vi "ORP电极校准.vi"() -> ()   [LabVIEW 2016, in "斯坦道多参数.lvlib"]
uses:
  <vilib>/Utility/miscctls.llb/LVPointTypeDef.ctl
  <vilib>/Analysis/NI_AALBase.lvlib
  <vilib>/Utility/config.llb/NI_LVConfig.lvlib
panel:
  in  "刷新按钮":bool
  out "第二点信号值":dbl
  out "第一点信号值":dbl
  out "通讯状态":string
  out "温度":dbl format="%#.2f"
  out "当前信号值":dbl caption="信号值" format="%#.2f"
  in  "校准停止":bool
  in  "校准启动":bool
  out "波形图表":dbl(graph) caption="历史曲线"
  out "第二点校准值":dbl
  out "第一点校准值":dbl
  in  "校准模式":u16(ring) items=["单点校准"]
  out "提示":string
  out "最小值":sgl format="%#.2f"
  out "最大值":sgl format="%#.2f"
  out "mean":dbl caption="均值" format="%#.2f"
  out "standard deviation":dbl caption="标准差" format="%#.2f"
  out "变异系数":dbl format="%#.6f"
  in  "标液1":dbl
  out "当前读取值":dbl caption="测量值" format="%#.2f"
  out "ORP偏移修正值":dbl format="%#.2f"
  # "ORP电极设定"
  # "请选择校准模式:"
  # "℃"
  # "mV"
  # "mV"
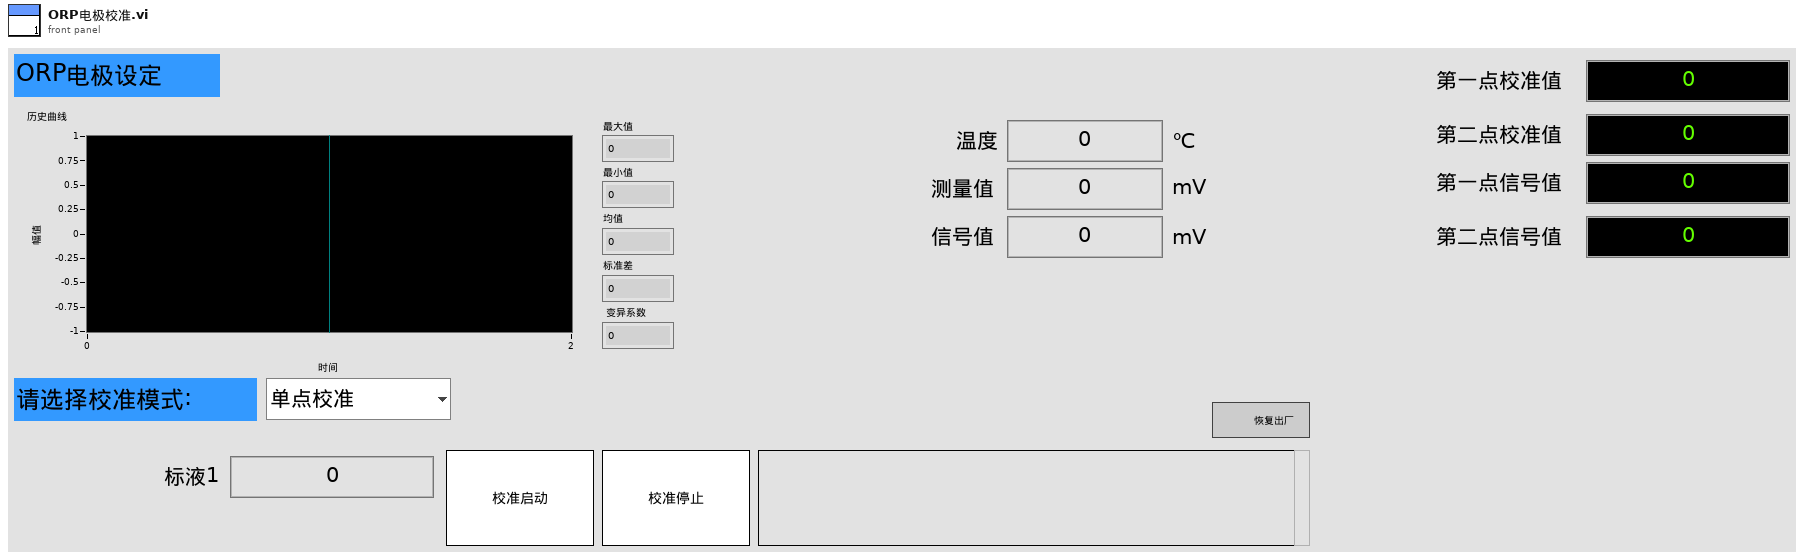
[diagram p1: front panel]
types:
  T1 = typedef "LVPointTypeDef.ctl" = cluster{"Horizontal":i16, "Vertical":i16}
  T2 = typedef "NI_LVConfig.lvlib/Config Data RefNum.ctl" = refnum<k1>
  T3 = cluster{"电极状态标志":u16, "电极型号标志":u16, "测量值":sgl, "温度测量值":sgl, "信号值":sgl, "温度信号值":sgl, "000AH_NC":sgl, "偏移修正值":sgl, "温度偏移修正值":sgl, "手动温度补偿值":sgl, "命令滤波设定":u16, "温度模式":enum16{"ATC", "MTC"}, "生产批次":u16, "传感器序号":u16, "串口地址":u16, "串口波特率":enum16{"9600", "19200", "115200"}, "串口校验位":enum16{"NONE", "ODD", "EVEN"}, "串口停止位":enum16{"1bit", "2bit"}}
  T4 = enum8{"Enabled", "Disabled", "Disabled and Grayed Out"}
  T5 = cluster{"ph":bool, "DO":bool, "Cond":bool, "Turb":bool, "叶绿素a":bool, "藻密度":bool, "ORP":bool}
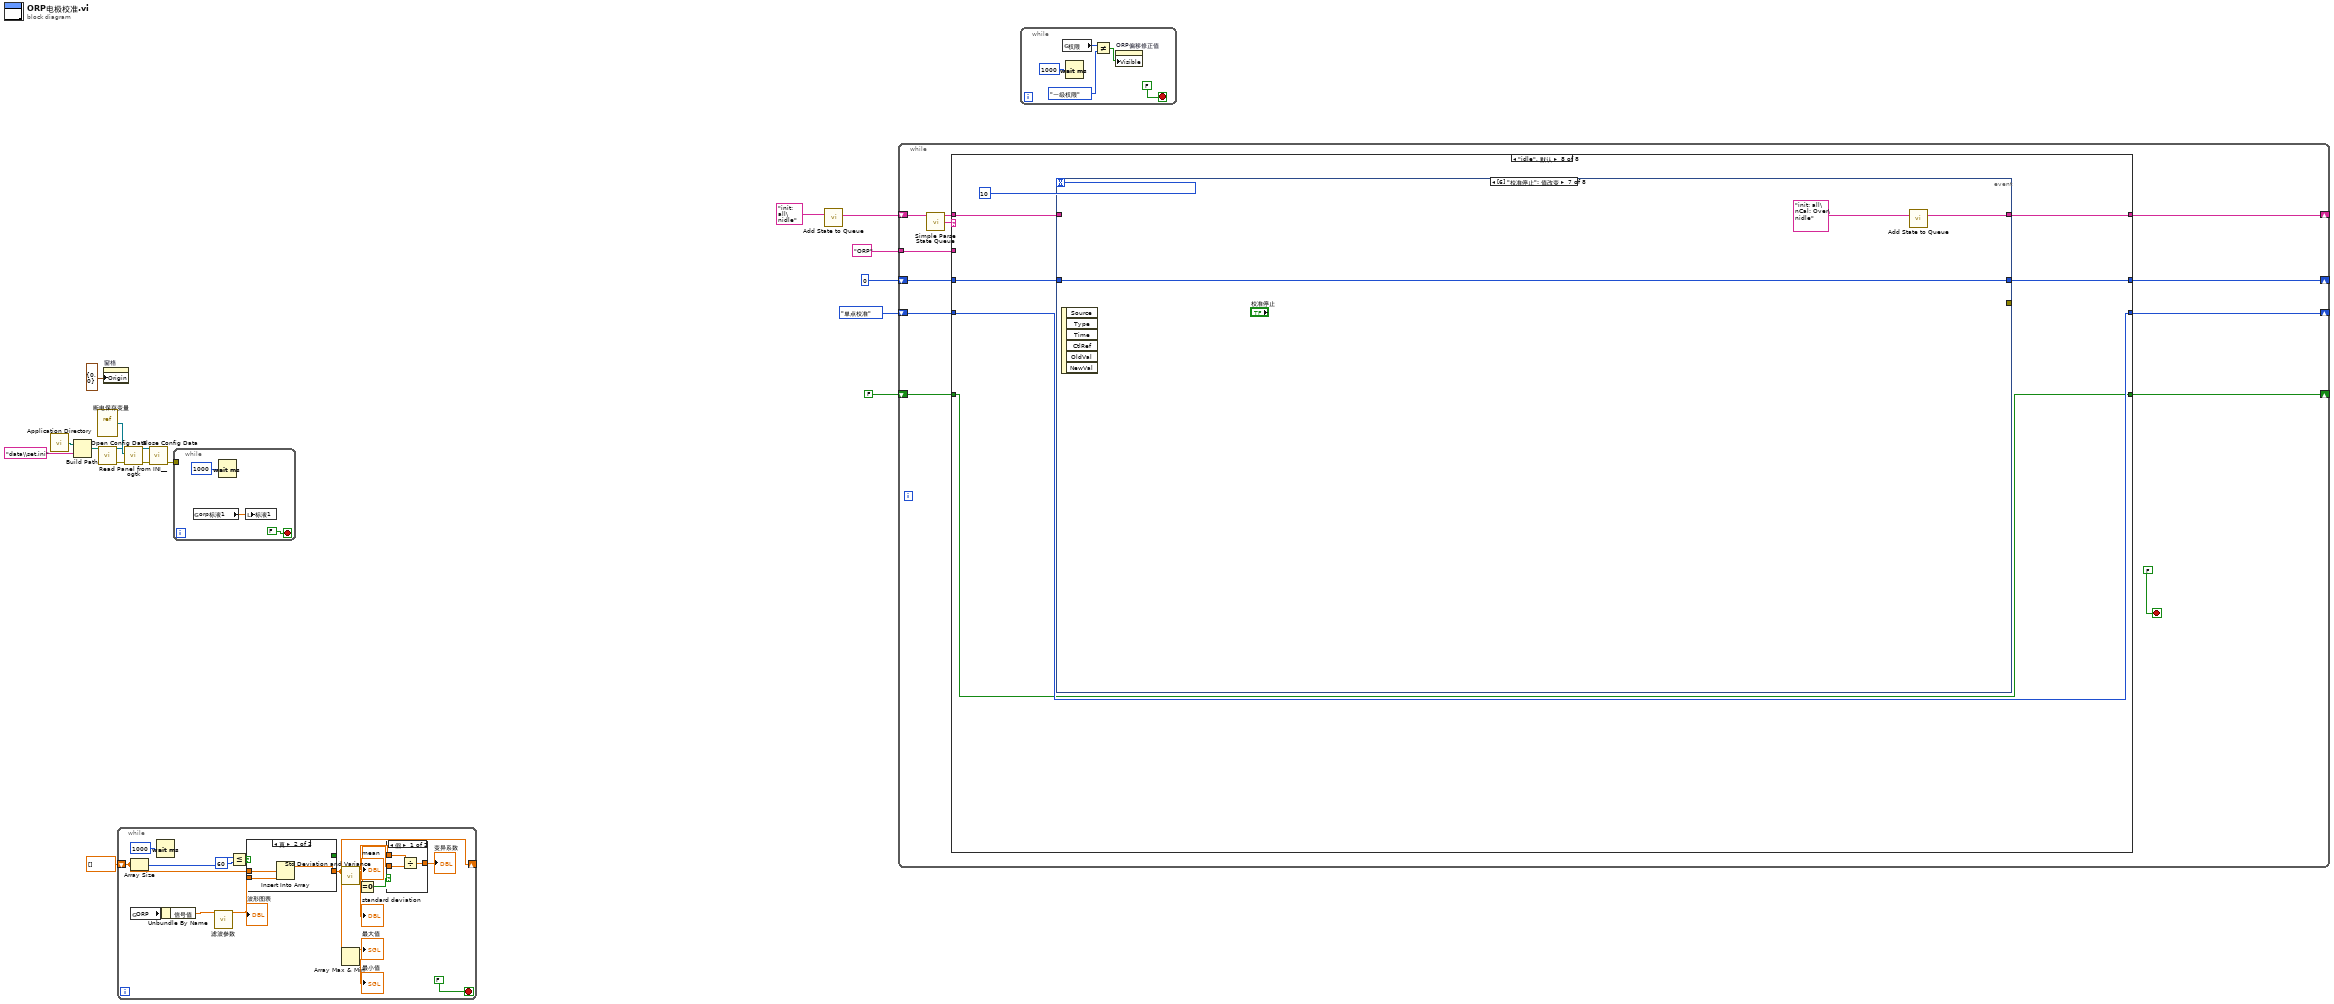
[diagram p0: block diagram]
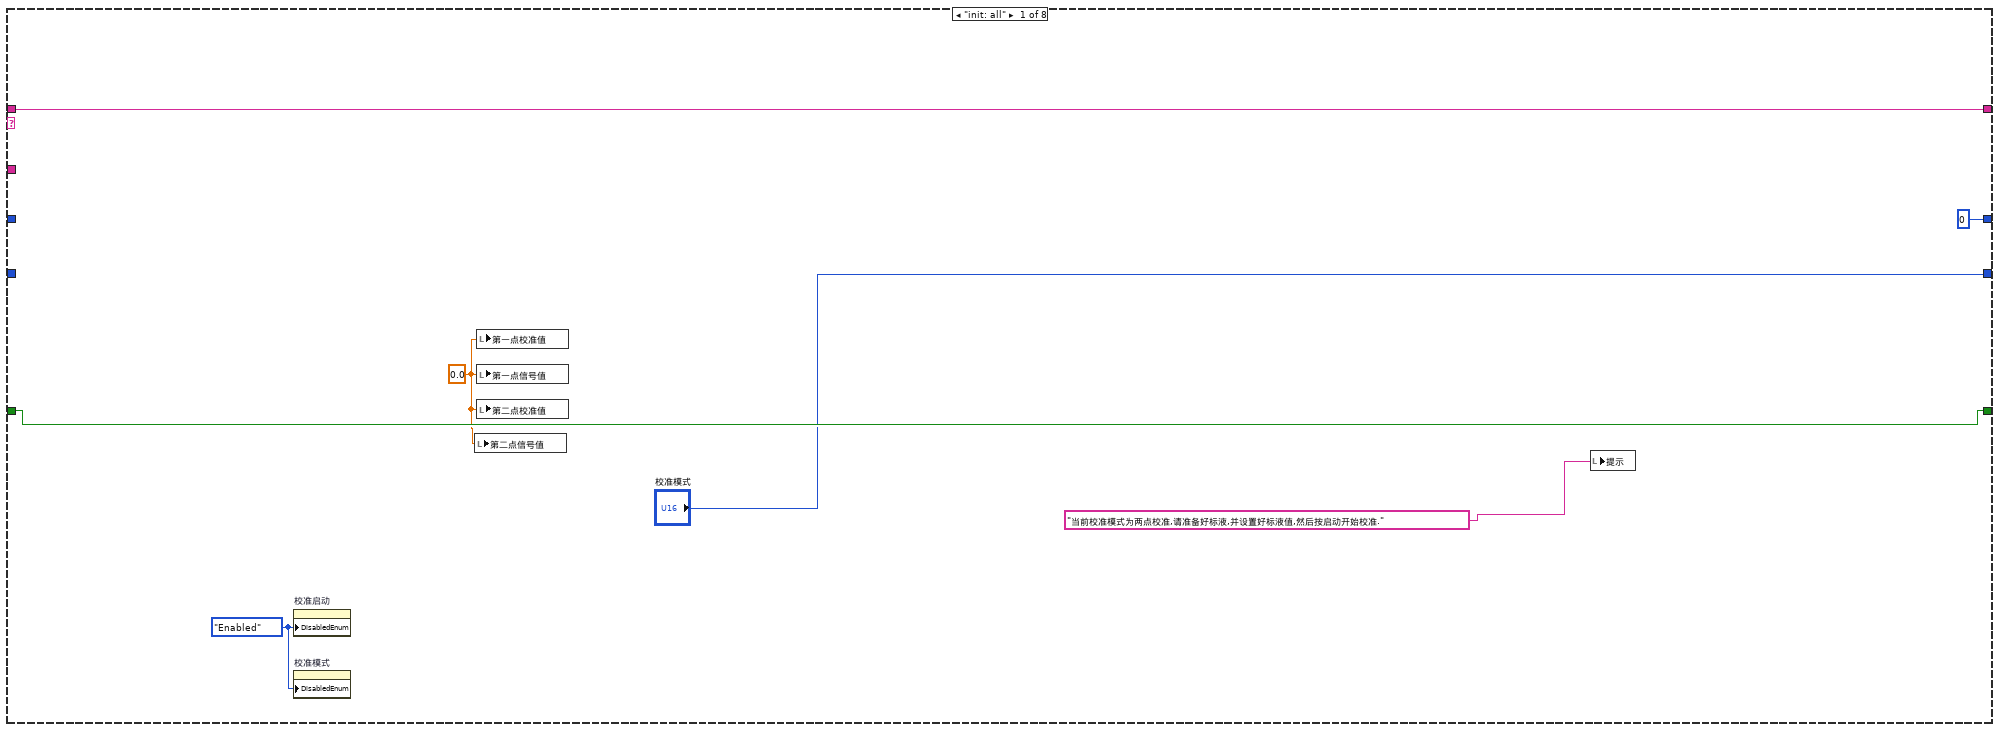
[diagram p2: hidden frame]
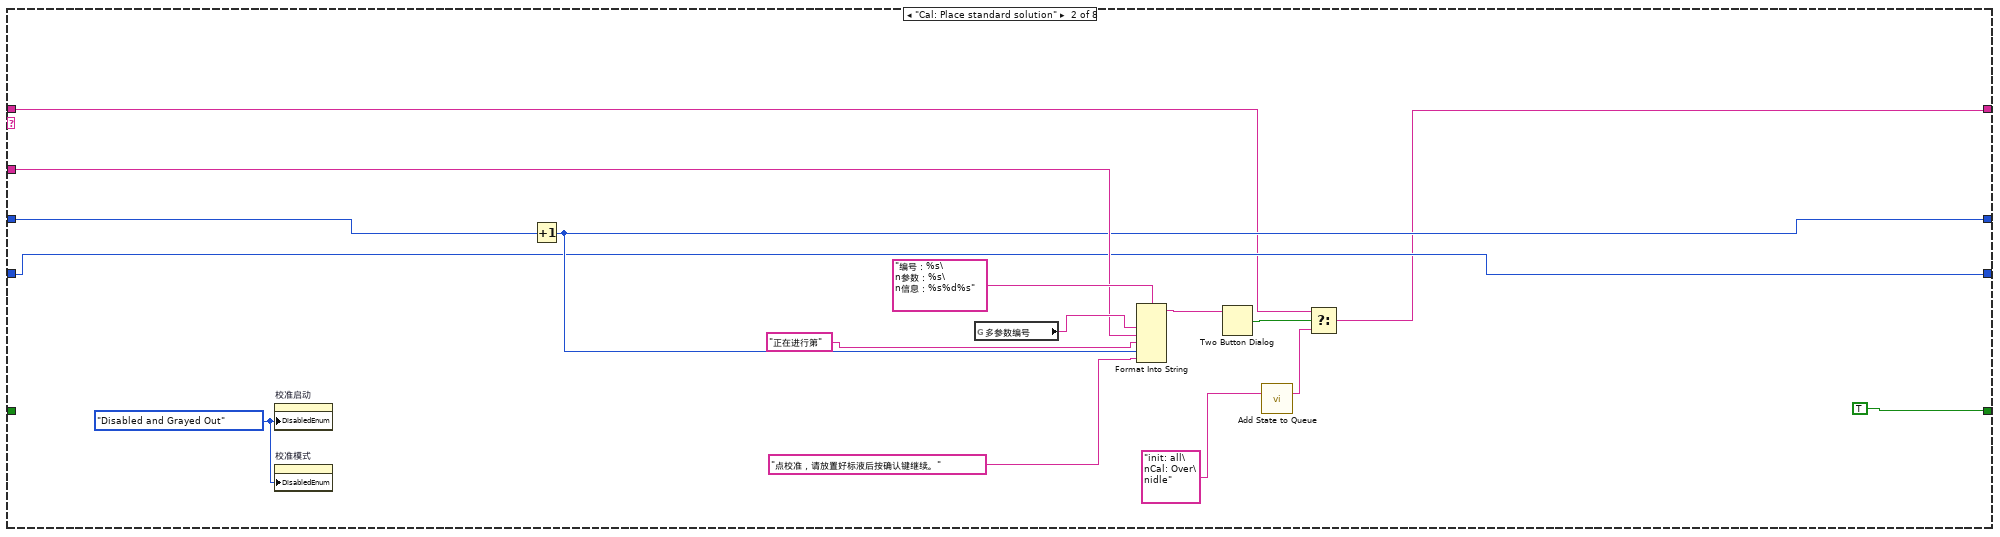
[diagram p3: hidden frame]
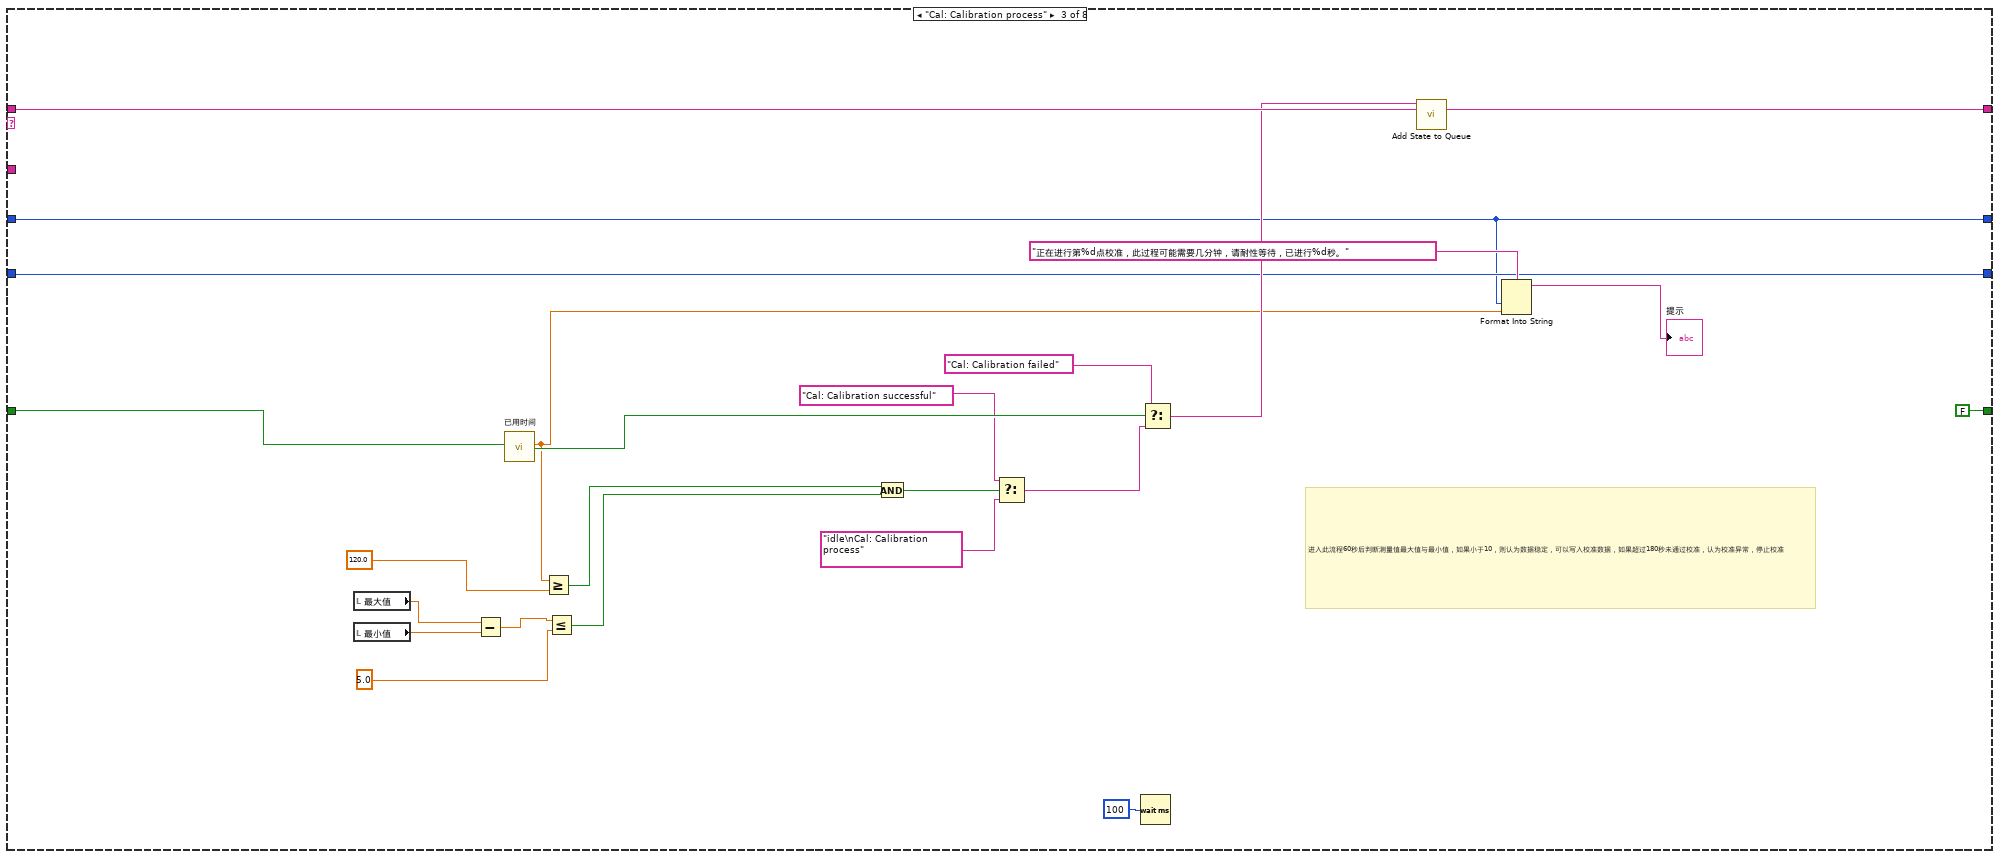
[diagram p4: hidden frame]
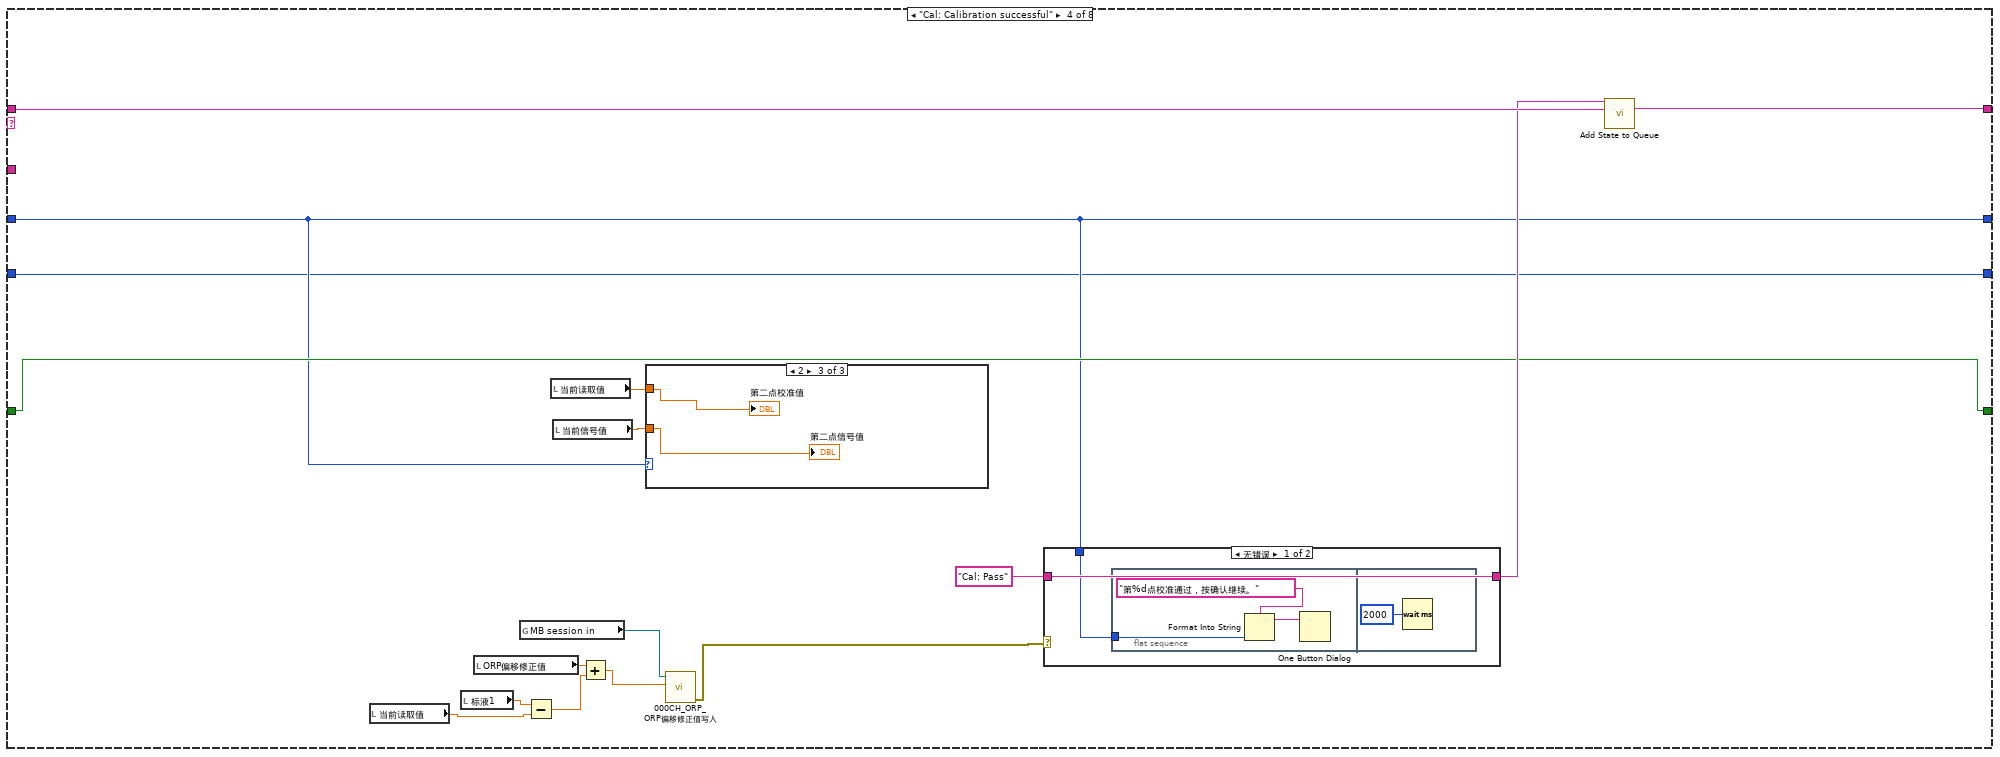
[diagram p5: hidden frame]
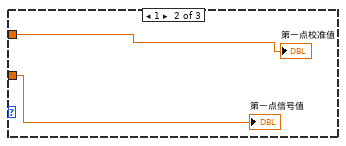
[diagram p7: hidden frame]
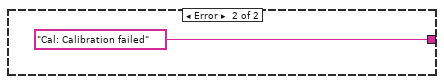
[diagram p8: hidden frame]
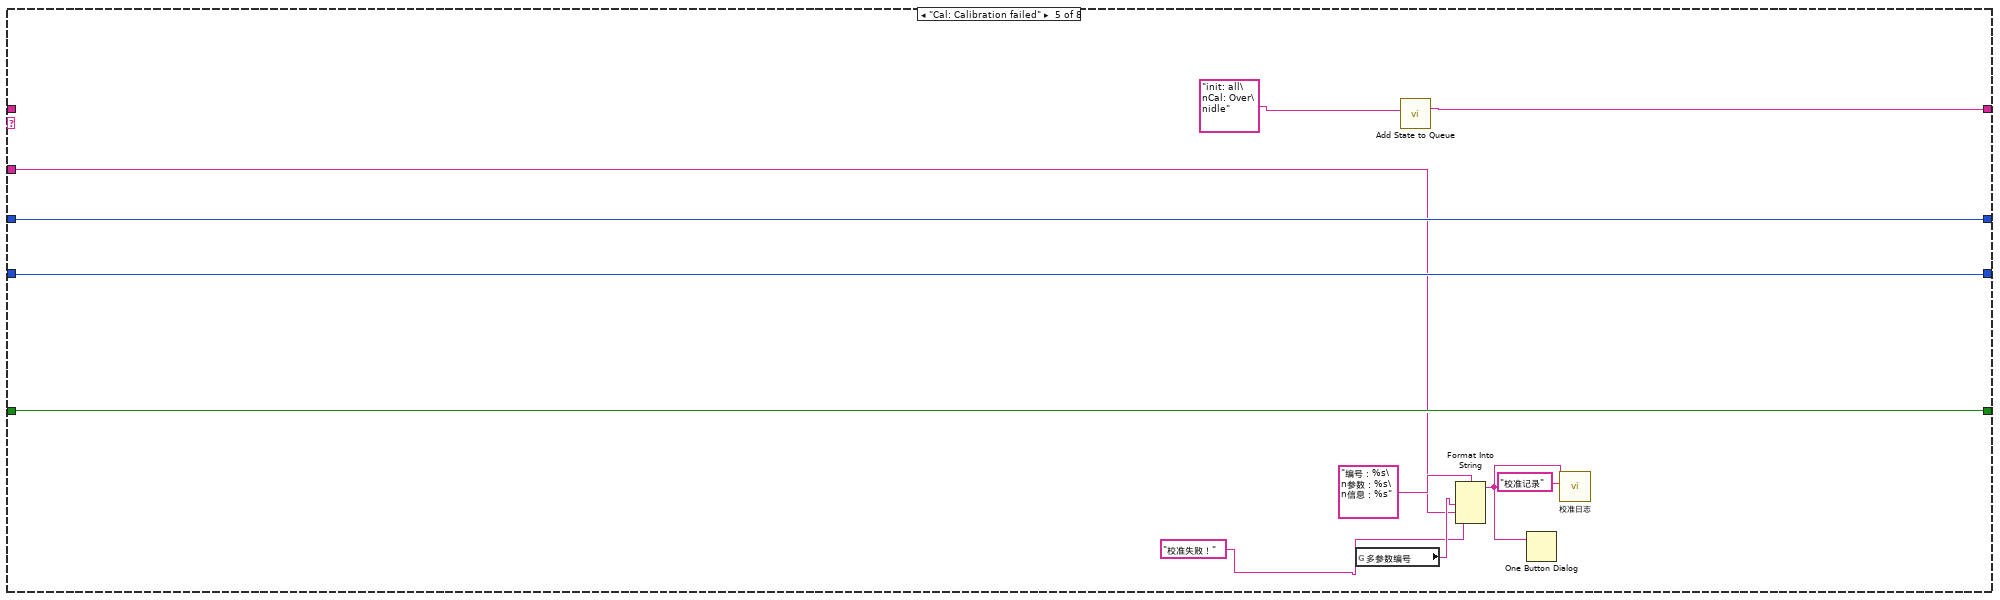
[diagram p9: hidden frame]
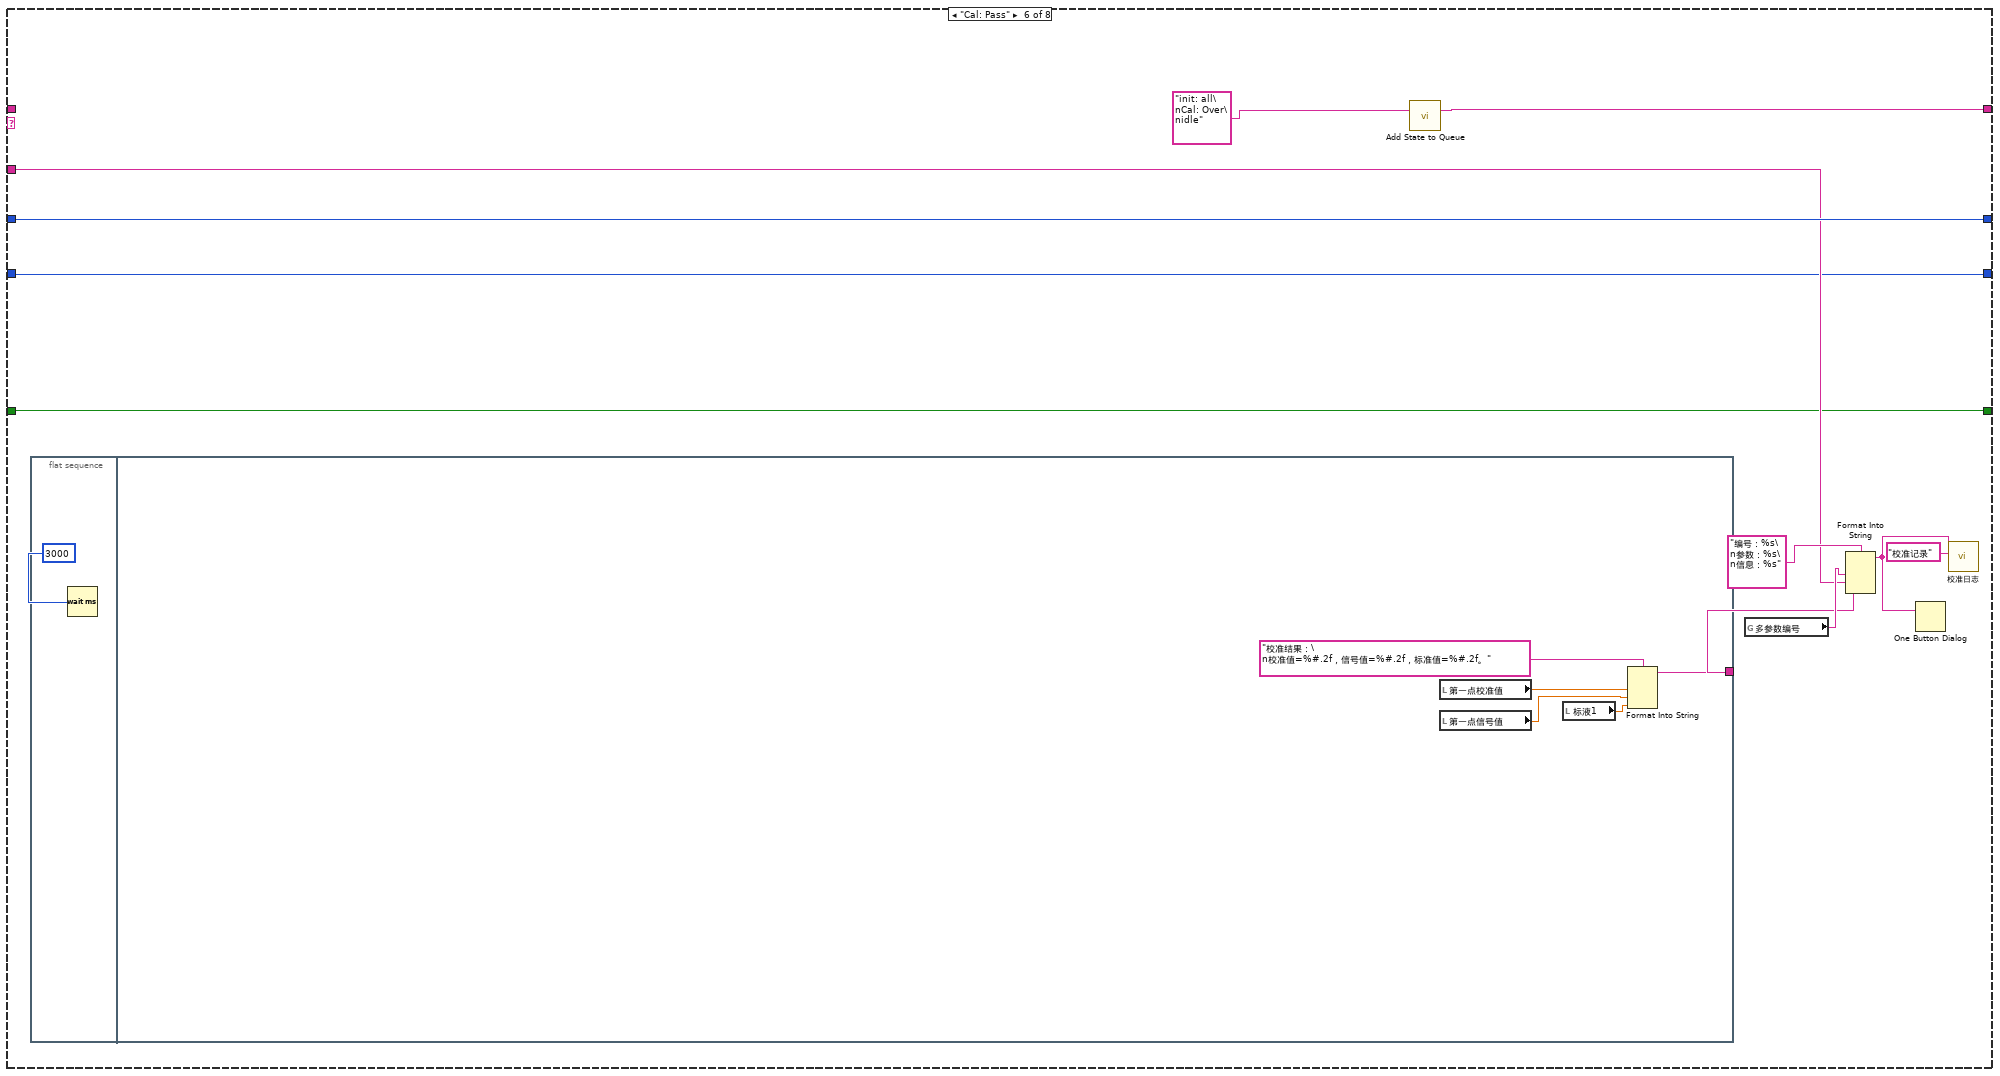
[diagram p10: hidden frame]
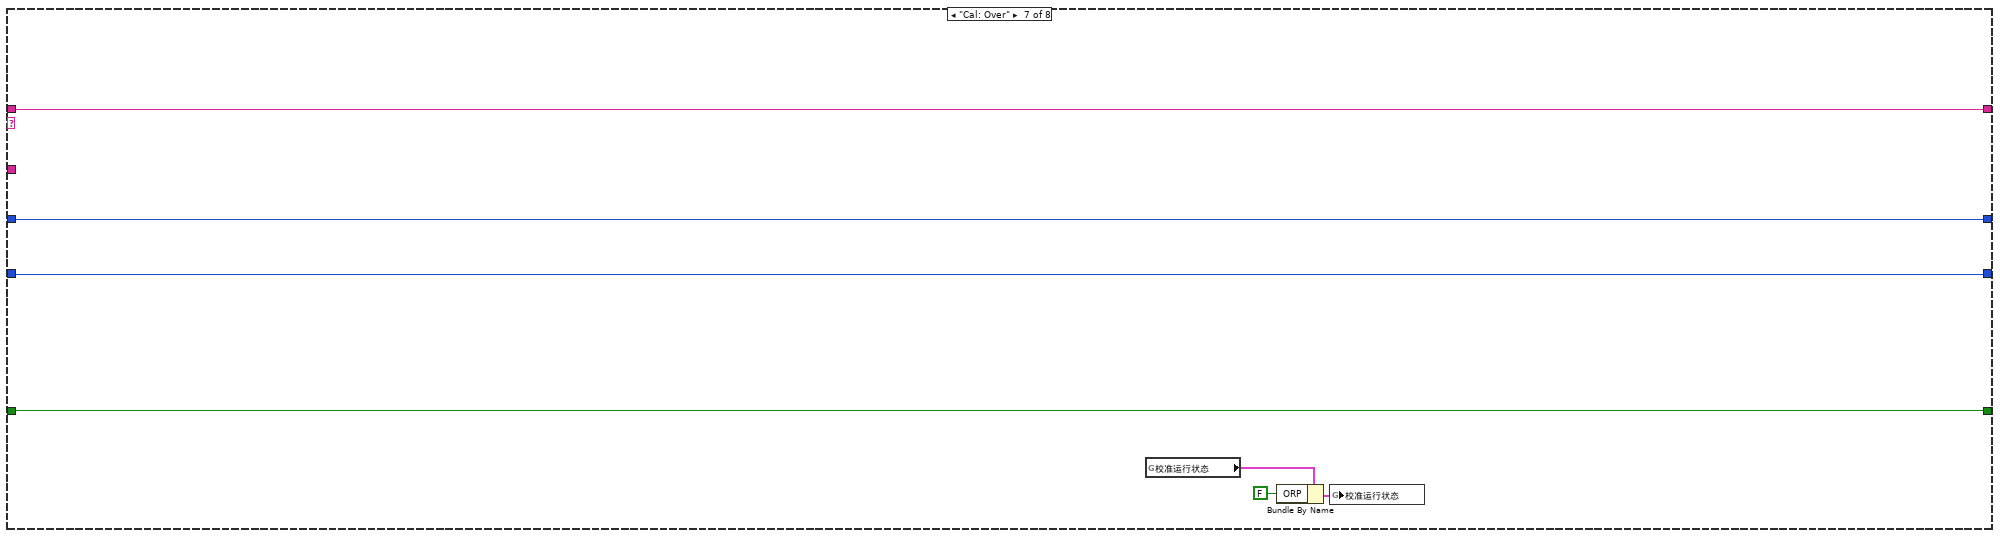
[diagram p11: hidden frame]
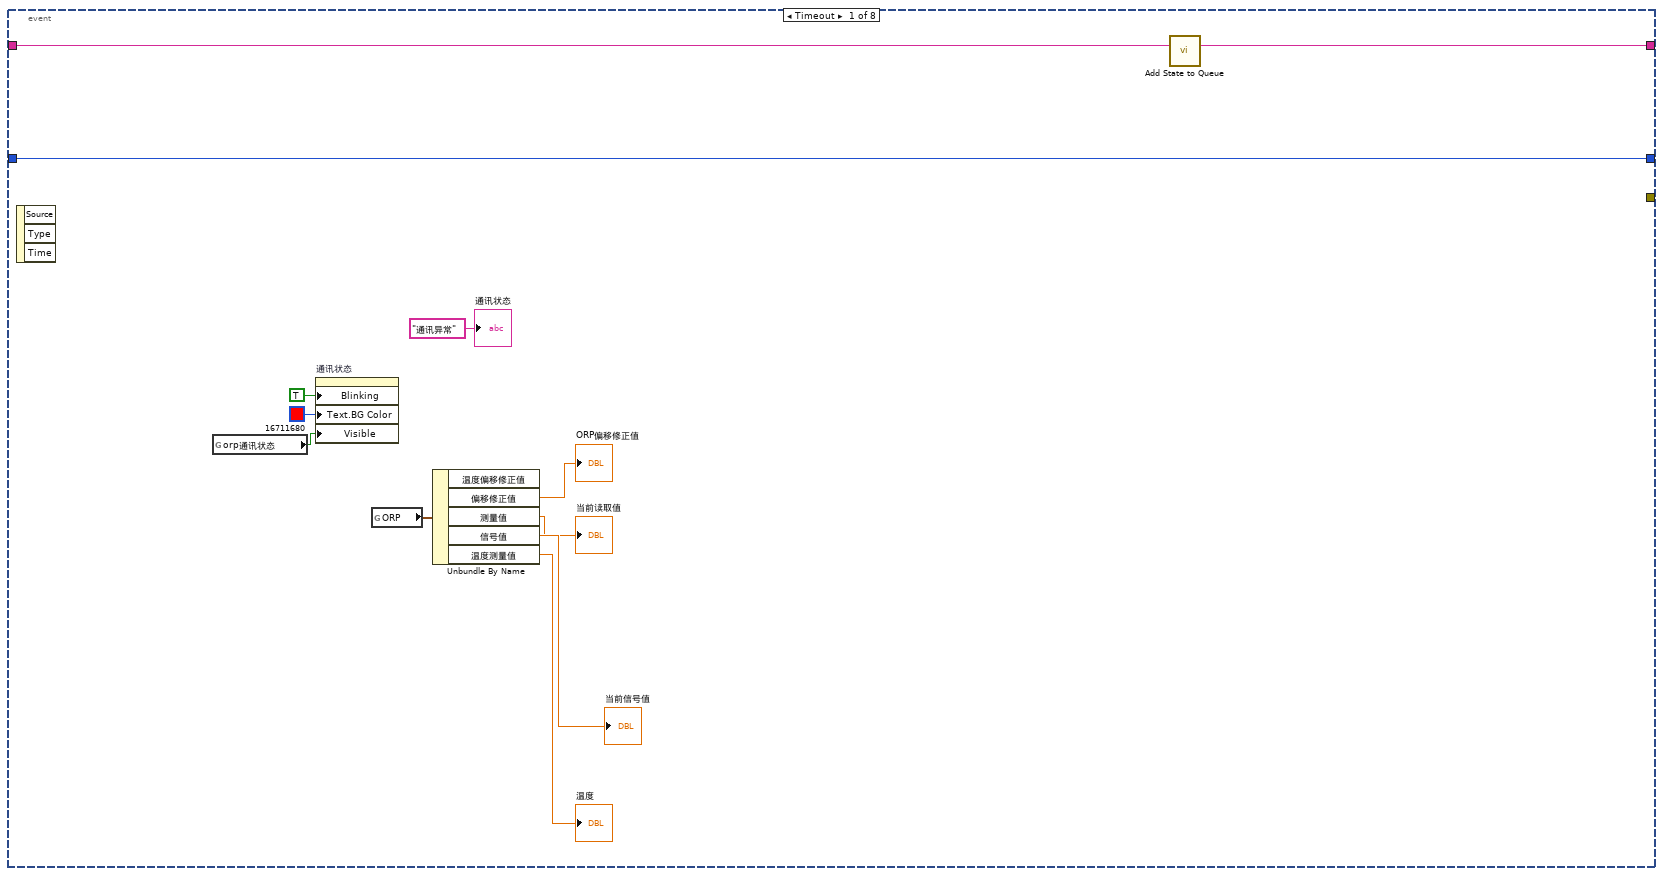
[diagram p12: hidden frame]
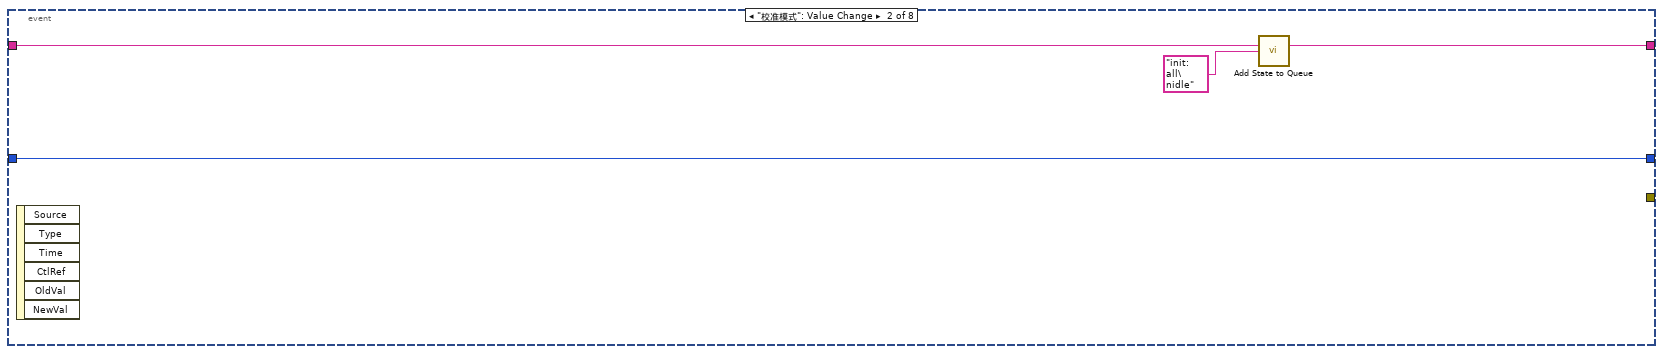
[diagram p13: hidden frame]
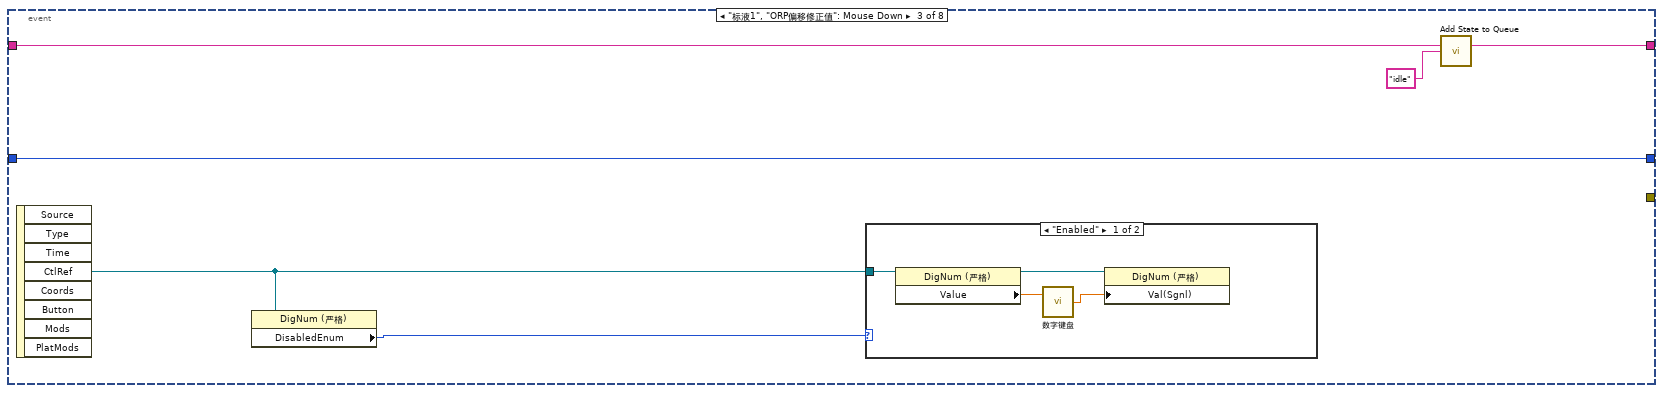
[diagram p14: hidden frame]
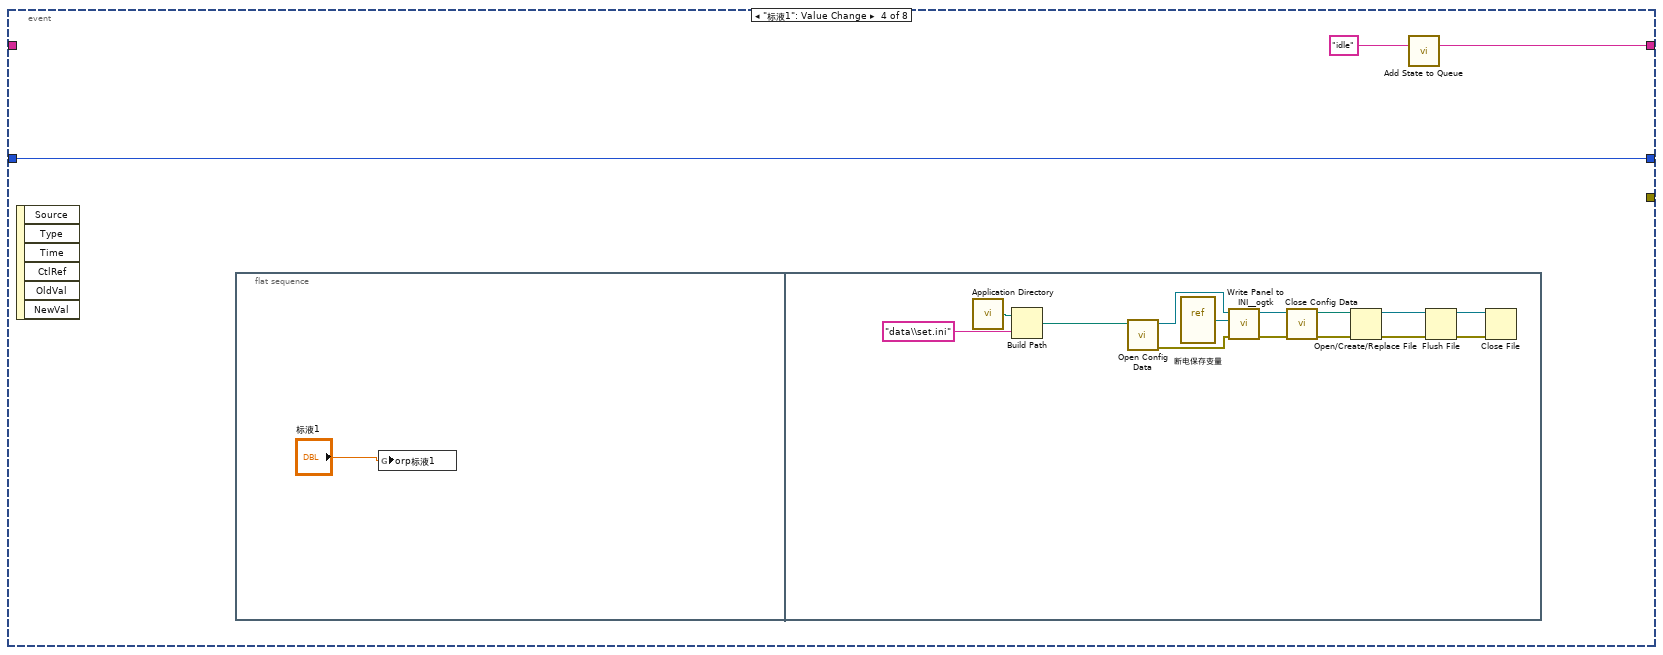
[diagram p16: hidden frame]
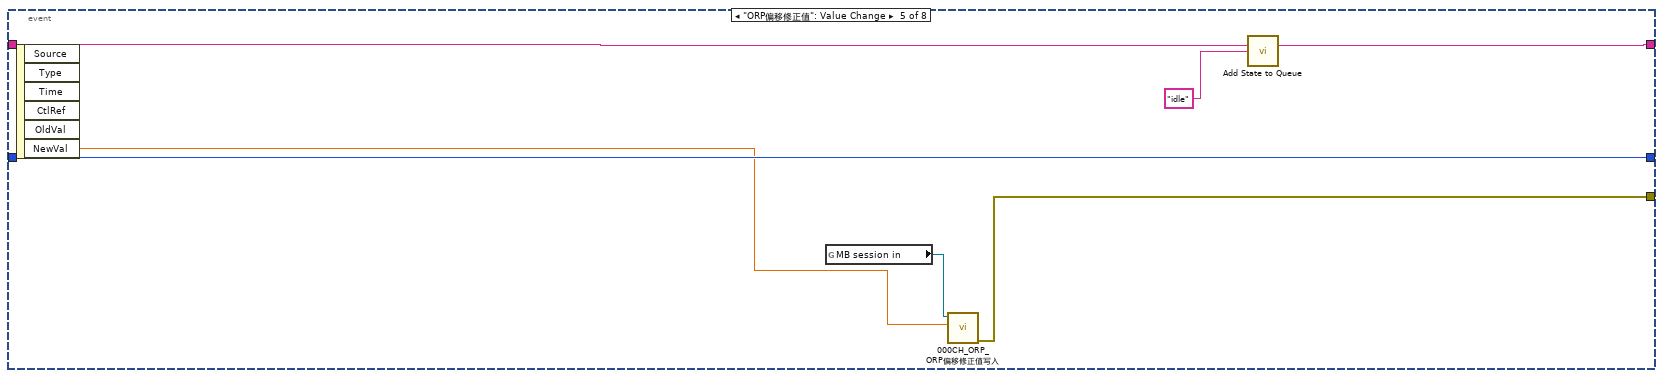
[diagram p17: hidden frame]
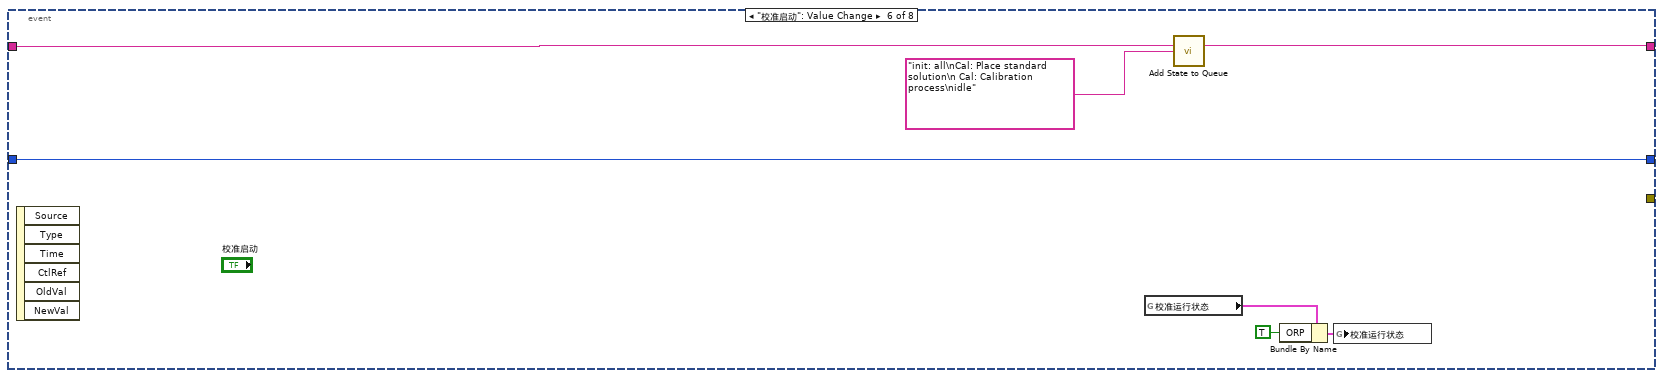
[diagram p18: hidden frame]
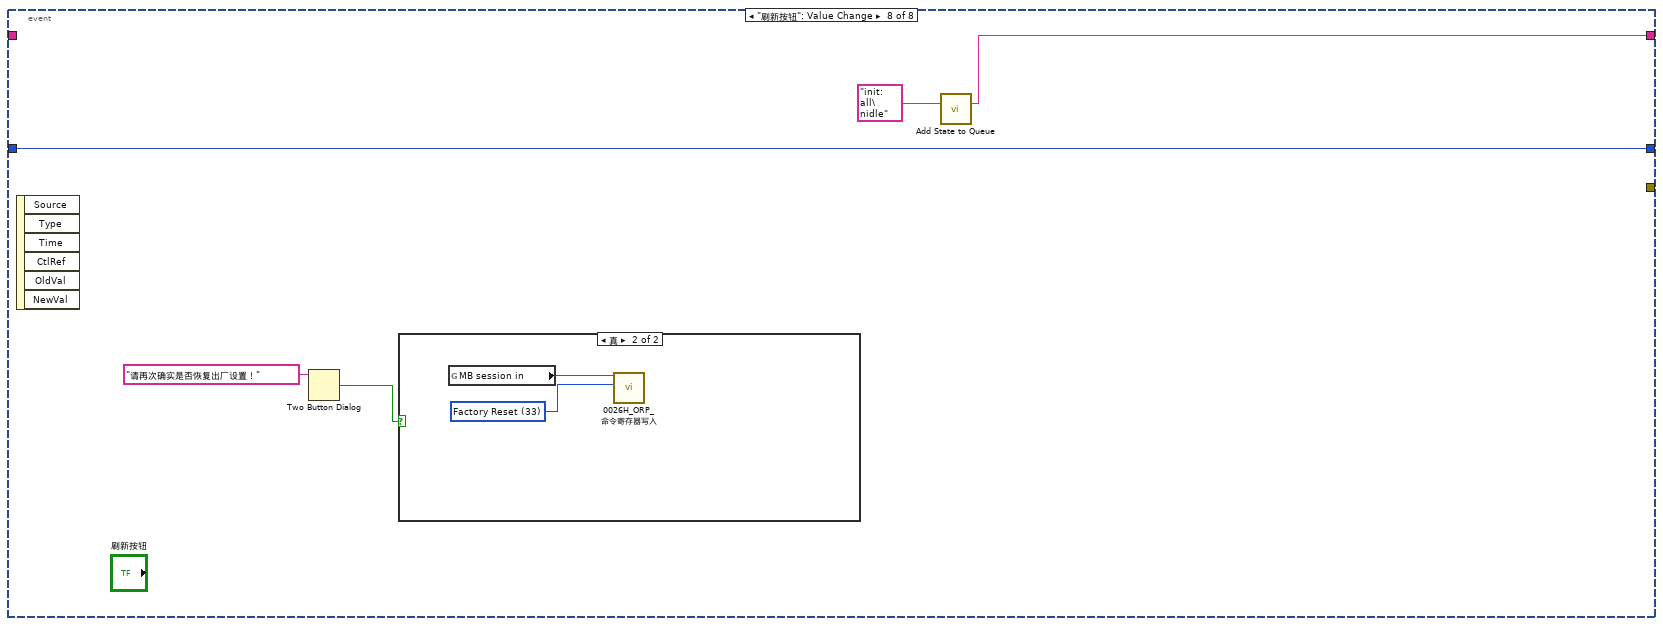
[diagram p19: hidden frame]
diagram:
  n1 = call <vilib>:"Application Directory.vi"() -> ("Application Directory"=w6:path)
  n2 = Build Path(base path=w6, name or relative path="data\\set.ini" ("名称或相对路径")) -> (appended path=w7:path)
  n3 = vi-ref "断电保存变量.vi"() -> (w9:refnum<vi>)
  n4 = call <vilib>:"Open Config Data.vi"("configuration file path"=w7) -> ("error out"=w3:errorcluster, "refnum"=w2:T2)  [unwired: 8 in, 1 out]
  n5 = property on="窗格" class="Pane"("Origin"=T1 {"Horizontal"=0, "Vertical"=0} ("原点")) -> ()  [unwired: 2 in, 2 out]
  n6 = while {
    shift-right: [w22] -> _
    shift-left: sgl[] [] -> [w29]
    stop <- FALSE stop-if-true
    n7 = Array Size(array=w29) -> (size(s)=w31:i32)
    n8 = global read "国弘过程全局变量.vi" "ORP"() -> (w23:T3)
    n9 = Wait (ms)(milliseconds to wait=u32 1000 ("等待时间（毫秒）")) -> ()  [unwired: 1 out]
    n10 = Unbundle By Name(w23) -> ("信号值"=w19:sgl)
    n11 = call "滤波参数.vi"("x"=w19) -> ("mode"=w18:dbl)  [unwired: 10 in]
    "波形图表" <- w18
    n12 = Less Or Equal?(x=w31, y=60) -> (x <= y?=w30:bool)
    n13 = case shown="真" w30 {
      tunnel: w29 -> [w42 w45]
      tunnel: w18 -> [w40 w44]
      tunnel: [w38 w43] -> w22
      tunnel: [TRUE _] -> _
      frame False {
        n14 = Replace Array Subset(array=w42, new element=w40) -> (w41:sgl[])  [unwired: 1 in]
        n15 = Rotate 1D Array(1:w41, 2:-1 ("n")) -> (0:w38:sgl[])
      }
      frame True {
        n16 = Insert Into Array(array=w45, new element=w44) -> (w43:sgl[])  [unwired: 1 in]
      }
    }
    n17 = call <vilib>:"Std Deviation and Variance.vi"("X"=w22) -> ("mean"=w27:dbl, "standard deviation"=w26:dbl)  [unwired: 1 in, 1 out]
    "mean" <- w27
    "standard deviation" <- w26
    n18 = Array Max & Min(array=w22) -> (max value=→"最大值":sgl, min value=→"最小值":sgl)  [unwired: 2 out]
    n19 = Equal To 0?(x=w27) -> (x = 0?=w28:bool)
    n20 = case shown="假" w28 {
      tunnel: w26 -> [w36 _]
      tunnel: [w35 _] -> w25
      tunnel: w27 -> [w34 _]
      frame False {
        n21 = Divide(x=w36, y=w34) -> (x/y=w35:dbl)
      }
      frame True {
      }
    }
    "变异系数" <- w25
  }
  n22 = call <userlib>:"Read Panel from INI__ogtk.vi"("error in (no error)"=w3, "VI ref"=w9, "refnum"=w2) -> ("error out"=w5:errorcluster, "refnum out"=w4:T2)  [unwired: 7 in]
  n23 = call <vilib>:"Close Config Data.vi"("error in (no error)"=w5, "refnum"=w4) -> ("error out"=w1:errorcluster)  [unwired: 8 in, 1 out]
  n24 = while {
    tunnel: w1 -> [_]
    stop <- FALSE stop-if-true
    n25 = global read "断电保存变量.vi" "orp标液1"() -> (w46:dbl)
    n26 = Wait (ms)(milliseconds to wait=u32 1000 ("等待时间（毫秒）")) -> ()  [unwired: 1 out]
    n27 = local write "标液1"(w46) -> ()
  }
  n28 = call "Add State to Queue.vi"("State(s) In (\"\")"="init: all\nidle" ("State(s) In (\"\")")) -> ("States Out"=w14:string)  [unwired: 14 in]
  n29 = while {
    shift-right: [w56] -> _
    shift-left: w14 -> [w60]
    shift-right: [w53] -> _
    shift-left: 0 -> [w55]
    tunnel: "ORP" ("State(s) In (\"\")") -> [w54]
    shift-right: [w51] -> _
    shift-left: enum16{"单点校准"}."单点校准" ("校准模式") -> [w52]
    shift-right: [w49] -> _
    shift-left: FALSE -> [w50]
    stop <- FALSE stop-if-true
    n30 = call "Simple Parse State Queue.vi"("State Queue"=w60) -> ("Remain States"=w57:string, "Next State"=w58:string)  [unwired: 13 in]
    n31 = case shown="\"idle\", 默认" w58 {
      tunnel: w57 -> [w67 w71 w102 w122 _ _ w166 w176]
      tunnel: [w67 w70 w101 w121 w142 w147 w166 w175] -> w56
      tunnel: w55 -> [_ w79 w86 w116 w145 w156 w163 w173]
      tunnel: w54 -> [_ w80 _ _ w136 w152 _ _]
      tunnel: [0 w77 w86 w116 w145 w156 w163 w174] -> w53
      tunnel: w52 -> [_ w76 w87 w115 w144 w148 w164 w172]
      tunnel: ["校准模式" w76 w87 w115 w144 w148 w164 w172] -> w51
      tunnel: w50 -> [w64 _ w89 w117 w143 w151 w165 w170]
      tunnel: [w64 TRUE FALSE w117 w143 w151 w165 w170] -> w49
      frame "init: all" {
        w62 = T4."Enabled" ("禁用")
        w61 = 0.0 ("第一点校准值")
        n32 = property on="校准启动" class="Bool"("DisabledEnum"=w62) -> ()  [unwired: 2 in, 2 out]
        n33 = property on="校准模式" class="Ring (严格)"("DisabledEnum"=w62) -> ()  [unwired: 2 in, 2 out]
        n34 = local write "第二点信号值"(w61) -> ()
        n35 = local write "第一点校准值"(w61) -> ()
        n36 = local write "第一点信号值"(w61) -> ()
        n37 = local write "第二点校准值"(w61) -> ()
        n38 = local write "提示"("当前校准模式为两点校准,请准备好标液,并设置好标液值,然后按启动开始校准." ("提示")) -> ()
      }
      frame "Cal: Place standard solution" {
        w69 = T4."Disabled and Grayed Out" ("禁用")
        n39 = property on="校准启动" class="Bool"("DisabledEnum"=w69) -> ()  [unwired: 2 in, 2 out]
        n40 = property on="校准模式" class="Ring (严格)"("DisabledEnum"=w69) -> ()  [unwired: 2 in, 2 out]
        n41 = Increment(x=w79) -> (x+1=w77:i32)
        n42 = global read "多参数全局变量.vi" "多参数编号"() -> (w82:string)
        n43 = Format Into String(format string="编号：%s\n参数：%s\n信息：%s%d%s" ("格式字符串"), w82, w80, "正在进行第" ("消息"), w77, "点校准，请放置好标液后按确认键继续。" ("消息")) -> (resulting string=w74:string)  [unwired: 2 in, 1 out]
        n44 = Two Button Dialog(message=w74) -> (T button?=w73:bool)  [unwired: 2 in]
        n45 = call "Add State to Queue.vi"("State(s) In (\"\")"="init: all\nCal: Over\nidle" ("State(s) In (\"\")")) -> ("States Out"=w72:string)  [unwired: 14 in]
        n46 = Select(t=w71, s=w73, f=w72) -> (s? t:f=w70:string)
      }
      frame "Cal: Calibration process" {
        # "进入此流程60秒后判断测量值最大值与最小值，如果小于10，则认为数据稳定，可以写入校准数据，如果超过180秒未通过校准，认为校准异常，停止校准"
        n47 = local read "最大值"() -> (w106:sgl)
        n48 = local read "最小值"() -> (w105:sgl)
        n49 = Subtract(x=w106, y=w105) -> (x-y=w107:sgl)
        n50 = call "已用时间"("Reset"=w89) -> ("Elapsed Time (s)"=w85:dbl, "Time has Elapsed"=w103:bool)  [unwired: 11 in, 6 out]
        n51 = Greater Or Equal?(x=w85, y=120.0) -> (x >= y?=w98:bool)
        n52 = Less Or Equal?(x=w107, y=5.0) -> (x <= y?=w94:bool)
        n53 = And(x=w98, y=w94) -> (x .and. y?=w95:bool)
        n54 = Select(t="Cal: Calibration successful" ("State(s) In (\"\")"), s=w95, f="idle\nCal: Calibration process" ("State(s) In (\"\")")) -> (s? t:f=w93:string)
        n55 = Wait (ms)(milliseconds to wait=u32 100 ("等待时间（毫秒）")) -> ()  [unwired: 1 out]
        n56 = Select(t="Cal: Calibration failed" ("State(s) In (\"\")"), s=w103, f=w93) -> (s? t:f=w92:string)
        n57 = call "Add State to Queue.vi"("State(s) In Front (\"\")"=w92, "State(s) In (\"\")"=w102) -> ("States Out"=w101:string)  [unwired: 13 in]
        n58 = Format Into String(format string="正在进行第%d点校准，此过程可能需要几分钟，请耐性等待，已进行%d秒。" ("格式字符串"), w86, w85) -> (resulting string=→"提示":string)  [unwired: 2 in, 1 out]
      }
      frame "Cal: Calibration successful" {
        n59 = local read "当前读取值"() -> (w111:dbl)
        n60 = local read "标液1"() -> (w114:dbl)
        n61 = local read "ORP偏移修正值"() -> (w112:dbl)
        n62 = global read "多参数全局变量.vi" "MB session in"() -> (w110:refnum<class "MB_Master.lvclass">)
        n63 = Subtract(x=w114, y=w111) -> (x-y=w113:dbl)
        n64 = local read "当前读取值"() -> (w118:dbl)
        n65 = local read "当前信号值"() -> (w119:dbl)
        n66 = Add(x=w112, y=w113) -> (x+y=w109:dbl)
        n67 = case shown="2" w116 {
          tunnel: w119 -> [_ w125 w127]
          tunnel: w118 -> [_ w124 w126]
          frame 0, Default {
          }
          frame 1 {
            "第一点信号值" <- w125
            "第一点校准值" <- w124
          }
          frame 2 {
            "第二点信号值" <- w127
            "第二点校准值" <- w126
          }
        }
        n68 = call "000CH_ORP_ORP偏移修正值写入.vi"("数值"=w109, "MB session in"=w110) -> ("error out"=w108:errorcluster)  [unwired: 8 in, 1 out]
        n69 = case shown="无错误" w108 {
          tunnel: "Cal: Pass" ("State(s) In (\"\")") -> [w129 _]
          tunnel: [w129 "Cal: Calibration failed" ("State(s) In (\"\")")] -> w120
          tunnel: w116 -> [w128 _]
          frame No Error {
            n70 = flat-sequence {
              tunnel: w128 -> [w130]
              frame #0 {
                n71 = Format Into String(format string="第%d点校准通过，按确认继续。" ("格式字符串"), w130) -> (resulting string=w132:string)  [unwired: 2 in, 1 out]
                n72 = One Button Dialog(message=w132) -> ()  [unwired: 1 in, 1 out]
              }
              frame #1 {
                n73 = Wait (ms)(milliseconds to wait=u32 2000 ("等待时间（毫秒）")) -> ()  [unwired: 1 out]
              }
            }
          }
          frame Error {
          }
        }
        n74 = call "Add State to Queue.vi"("State(s) In Front (\"\")"=w120, "State(s) In (\"\")"=w122) -> ("States Out"=w121:string)  [unwired: 13 in]
      }
      frame "Cal: Calibration failed" {
        n75 = global read "多参数全局变量.vi" "多参数编号"() -> (w139:string)
        n76 = call "Add State to Queue.vi"("State(s) In (\"\")"="init: all\nCal: Over\nidle" ("State(s) In (\"\")")) -> ("States Out"=w142:string)  [unwired: 14 in]
        n77 = Format Into String(format string="编号：%s\n参数：%s\n信息：%s" ("格式字符串"), w139, w136, "校准失败！" ("消息")) -> (resulting string=w138:string)  [unwired: 2 in, 1 out]
        n78 = One Button Dialog(message=w138) -> ()  [unwired: 1 in, 1 out]
        n79 = call "校准日志.vi"("table"="校准记录", "日志信息"=w138) -> ()  [unwired: 9 in, 1 out]
      }
      frame "Cal: Pass" {
        n80 = flat-sequence {
          tunnel: [w162] -> w149
          frame #0 {
            n81 = Wait (ms)(milliseconds to wait=u32 3000 ("等待时间（毫秒）")) -> ()  [unwired: 1 out]
          }
          frame #1 {
            n82 = local read "第一点校准值"() -> (w161:dbl)
            n83 = local read "第一点信号值"() -> (w159:dbl)
            n84 = local read "标液1"() -> (w158:dbl)
            n85 = Format Into String(format string="校准结果：\n校准值=%#.2f，信号值=%#.2f，标准值=%#.2f。" ("提示"), w161, w159, w158) -> (resulting string=w162:string)  [unwired: 2 in, 1 out]
          }
        }
        n86 = call "Add State to Queue.vi"("State(s) In (\"\")"="init: all\nCal: Over\nidle" ("State(s) In (\"\")")) -> ("States Out"=w147:string)  [unwired: 14 in]
        n87 = global read "多参数全局变量.vi" "多参数编号"() -> (w153:string)
        n88 = Format Into String(format string="编号：%s\n参数：%s\n信息：%s" ("格式字符串"), w153, w152, w149) -> (resulting string=w150:string)  [unwired: 2 in, 1 out]
        n89 = One Button Dialog(message=w150) -> ()  [unwired: 1 in, 1 out]
        n90 = call "校准日志.vi"("table"="校准记录", "日志信息"=w150) -> ()  [unwired: 9 in, 1 out]
      }
      frame "Cal: Over" {
        n91 = global read "多参数全局变量.vi" "校准运行状态"() -> (w168:T5)
        n92 = Bundle By Name(cluster=w168, "ORP"=FALSE) -> (w169:T5)
        n93 = global write "多参数全局变量.vi" "校准运行状态"(w169) -> ()
      }
      frame "idle", Default {
        n94 = event shown="[6] \"校准停止\": 值改变" {
          selector: _ -> [_ _ _ _ _ _ _ _]
          dyn-events: _ -> [_ _ _ _ _ _ _ _]
          timeout: 10 -> [_ _ _ _ _ _ _ _]
          tunnel: [_ _ _ _ w222 _ _ _] -> _
          tunnel: w176 -> [w188 w192 w195 _ w227 w234 _ _]
          tunnel: [w187 w191 w197 w203 w226 w233 w236 w239] -> w175
          tunnel: [w186 w189 w198 w205 w225 w231 w237 w238] -> w174
          tunnel: w173 -> [w186 w189 w198 w205 w225 w231 w237 w238]
          event Timeout {
            n95 = event-data() -> ()  [unwired: 1 in, 3 out]
            n96 = global read "多参数全局变量.vi" "orp通讯状态"() -> (w184:bool)
            n97 = property on="通讯状态" class="Str"("Blinking"=TRUE ("闪烁"), "Text.BG Color"=u32 16711680, "Visible"=w184) -> ()  [unwired: 2 in, 2 out]
            n98 = global read "国弘过程全局变量.vi" "ORP"() -> (w177:T3)
            n99 = Unbundle By Name(w177) -> ("偏移修正值"=→"ORP偏移修正值":sgl, "测量值"=→"当前读取值":sgl, "信号值"=→"当前信号值":sgl, "温度测量值"=→"温度":sgl)  [unwired: 1 out]
            n100 = call "Add State to Queue.vi"("State(s) In (\"\")"=w188) -> ("States Out"=w187:string)  [unwired: 14 in]
            "通讯状态" <- "通讯异常" ("当前串口")
          }
          event "校准模式": Value Change {
            n101 = event-data() -> ()  [unwired: 1 in, 6 out]
            n102 = call "Add State to Queue.vi"("State(s) In (\"\")"=w192, "State(s) At Back (\"\")"="init: all\nidle" ("State(s) In (\"\")")) -> ("States Out"=w191:string)  [unwired: 13 in]
          }
          event "标液1", "ORP偏移修正值": Mouse Down {
            n103 = event-data() -> ("CtlRef"=w194:refnum<vi>)  [unwired: 1 in, 7 out]
            n104 = property class="DigNum (严格)"(reference=w194) -> ("DisabledEnum"=w193:T4)  [unwired: 1 in, 2 out]
            n105 = case shown="\"Enabled\"" w193 {
              tunnel: w194 -> [w202 _]
              frame "Enabled" {
                n106 = property class="DigNum (严格)"(reference=w202) -> (reference out=w199:refnum<vi>, "Value"=w200:dbl)  [unwired: 1 in, 1 out]
                n107 = call "数字键盘.vi"("OldNumber"=w200) -> ("NewNumber"=w201:dbl)  [unwired: 1 in]
                n108 = property class="DigNum (严格)"(reference=w199, "Val(Sgnl)"=w201) -> ()  [unwired: 1 in, 2 out]
              }
              frame "Disabled", Default {
              }
            }
            n109 = call "Add State to Queue.vi"("State(s) In (\"\")"=w195, "State(s) At Back (\"\")"="idle" ("State(s) In (\"\")")) -> ("States Out"=w197:string)  [unwired: 13 in]
          }
          event "标液1": Value Change {
            n110 = event-data() -> ()  [unwired: 1 in, 6 out]
            n111 = flat-sequence {
              frame #0 {
                n112 = global write "断电保存变量.vi" "orp标液1"("标液1") -> ()
              }
              frame #1 {
                n113 = call <vilib>:"Application Directory.vi"() -> ("Application Directory"=w216:path)
                n114 = Build Path(base path=w216, name or relative path="data\\set.ini" ("名称或相对路径")) -> (appended path=w215:path)
                n115 = call <vilib>:"Open Config Data.vi"("configuration file path"=w215) -> ("error out"=w219:errorcluster, "refnum"=w220:T2)  [unwired: 8 in, 1 out]
                n116 = vi-ref "断电保存变量.vi"() -> (w213:refnum<vi>)
                n117 = call <userlib>:"Write Panel to INI__ogtk.vi"("error in (no error)"=w219, "VI ref"=w213, "refnum"=w220) -> ("error out"=w217:errorcluster, "refnum out"=w218:T2)  [unwired: 7 in]
                n118 = call <vilib>:"Close Config Data.vi"("error in (no error)"=w217, "refnum"=w218) -> ("error out"=w209:errorcluster, "file path"=w210:path)  [unwired: 8 in]
                n119 = Open/Create/Replace File(file path (use dialog)=w210, error in=w209) -> (refnum out=w211:refnum<file>, error out=w212:errorcluster)  [unwired: 4 in, 1 out]
                n120 = Flush File(refnum=w211, error in=w212) -> (refnum out=w207:refnum<file>, error out=w208:errorcluster)
                n121 = Close File(refnum=w207, error in=w208) -> ()  [unwired: 2 out]
              }
            }
            n122 = call "Add State to Queue.vi"("State(s) In (\"\")"="idle" ("State(s) In (\"\")")) -> ("States Out"=w203:string)  [unwired: 14 in]
          }
          event "ORP偏移修正值": Value Change {
            n123 = event-data() -> ("NewVal"=w221:dbl)  [unwired: 1 in, 5 out]
            n124 = global read "多参数全局变量.vi" "MB session in"() -> (w223:refnum<class "MB_Master.lvclass">)
            n125 = call "000CH_ORP_ORP偏移修正值写入.vi"("数值"=w221, "MB session in"=w223) -> ("error out"=w222:errorcluster)  [unwired: 8 in, 1 out]
            n126 = call "Add State to Queue.vi"("State(s) In (\"\")"=w227, "State(s) At Back (\"\")"="idle" ("State(s) In (\"\")")) -> ("States Out"=w226:string)  [unwired: 13 in]
          }
          event "校准启动": Value Change {
            n127 = event-data() -> ()  [unwired: 1 in, 6 out]
            n128 = global read "多参数全局变量.vi" "校准运行状态"() -> (w229:T5)
            n129 = call "Add State to Queue.vi"("State(s) In (\"\")"=w234, "State(s) At Back (\"\")"="init: all\nCal: Place standard solution\n Cal: Calibration process\nidle" ("State(s) In (\"\")")) -> ("States Out"=w233:string)  [unwired: 13 in]
            n130 = Bundle By Name(cluster=w229, "ORP"=TRUE) -> (w230:T5)
            n131 = global write "多参数全局变量.vi" "校准运行状态"(w230) -> ()
          }
          event "校准停止": Value Change {
            n132 = event-data() -> ()  [unwired: 1 in, 6 out]
            n133 = call "Add State to Queue.vi"("State(s) In (\"\")"="init: all\nCal: Over\nidle" ("State(s) In (\"\")")) -> ("States Out"=w236:string)  [unwired: 14 in]
          }
          event "刷新按钮": Value Change {
            n134 = event-data() -> ()  [unwired: 1 in, 6 out]
            n135 = Two Button Dialog(message="请再次确实是否恢复出厂设置！" ("消息")) -> (T button?=w242:bool)  [unwired: 2 in]
            n136 = case shown="真" w242 {
              frame False {
              }
              frame True {
                w243 = u16 33 items=["Factory Reset"=33] ("数值")
                n137 = global read "多参数全局变量.vi" "MB session in"() -> (w244:refnum<class "MB_Master.lvclass">)
                n138 = call "0026H_ORP_命令寄存器写入.vi"("数值"=w243, "MB session in"=w244) -> ()  [unwired: 8 in, 2 out]
              }
            }
            n139 = call "Add State to Queue.vi"("State(s) In (\"\")"="init: all\nidle" ("State(s) In (\"\")")) -> ("States Out"=w239:string)  [unwired: 14 in]
          }
        }
      }
    }
  }
  n140 = while {
    stop <- FALSE stop-if-true
    n141 = global read "多参数全局变量.vi" "权限"() -> (w248:enum16{"一级权限", "二级权限", "三级权限"})
    n142 = Wait (ms)(milliseconds to wait=u32 1000 ("等待时间（毫秒）")) -> ()  [unwired: 1 out]
    n143 = Not Equal?(x=w248, y=enum16{"一级权限", "二级权限", "三级权限"}."一级权限") -> (x != y?=w246:bool)
    n144 = property on="ORP偏移修正值" class="DigNum (严格)"("Visible"=w246) -> ()  [unwired: 2 in, 2 out]
  }
